vi "newSubject.vi"(8 "error in (no error)":errorcluster, 11 "reference in":refnum<class "Subject Controller.lvclass">) -> (0 "error out":errorcluster, 3 "reference out":refnum<class "Subject Controller.lvclass">)   [LabVIEW 2015, in "Subject Controller.lvclass"]
uses:
  Subject Controller.lvclass
  File Controller_llb/File Controller.lvclass
  APP/subject_class/subject.lvclass
  APP/subject_class/phase.ctl
  APP/subject_class/resultsType.ctl
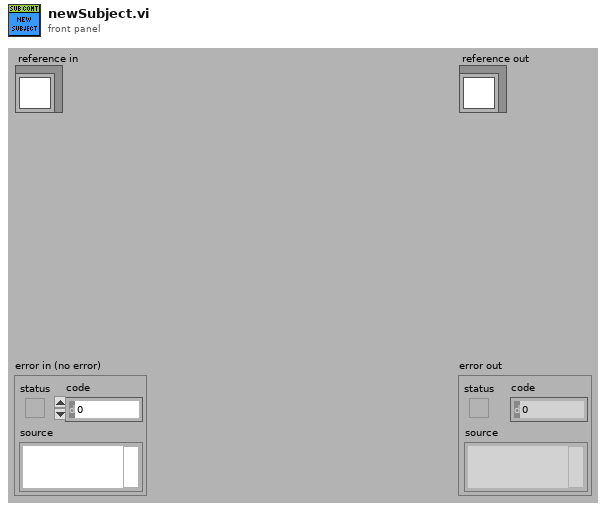
[diagram p1: front panel]
types:
  T1 = cluster{"Ve_warm":dbl[], "time_warm":dbl[], "name":string, "phase":dbl[], "VCO2":dbl[], "VO2":dbl[], "PetCO2":dbl[], "RQ":dbl[], "HR":dbl[], "Ve_warm_inter":dbl[], "time_warm_inter":dbl[], "Ve_exer":dbl[], "time_exer":dbl[], "Ve_exer_inter":dbl[], "time_exer_inter":dbl[], "Ve":dbl[], "time":dbl[], "Ve_exer_inter_filtered":dbl[], "Ve_warm_inter_filtered":dbl[]}
  T2 = typedef "Subject Controller.lvclass/ObjectAttributesRef.ctl" = refnum<data-value>
  T3 = typedef "Subject Controller.lvclass/ObjectAttributes.ctl" = cluster{"MyAttribute":dbl, "subject_controller_ref":refnum<class "Subject Controller.lvclass">, "file_controller_ref":refnum<class "File Controller.lvclass">, "subject_refs":refnum<class "subject.lvclass">[], "subjectIndex":i32, "file_type":T4}
  T4 = typedef "excelFile.lvclass/fileType.ctl" = enum16{"database", "CosmedTest"}
  T5 = typedef "subject.lvclass/resultsType.ctl" = enum16{"5L", "15%", "User Selection"}
  T6 = typedef "subject.lvclass/phase.ctl" = enum16{"warmUp", "userSelection", "Exercise"}
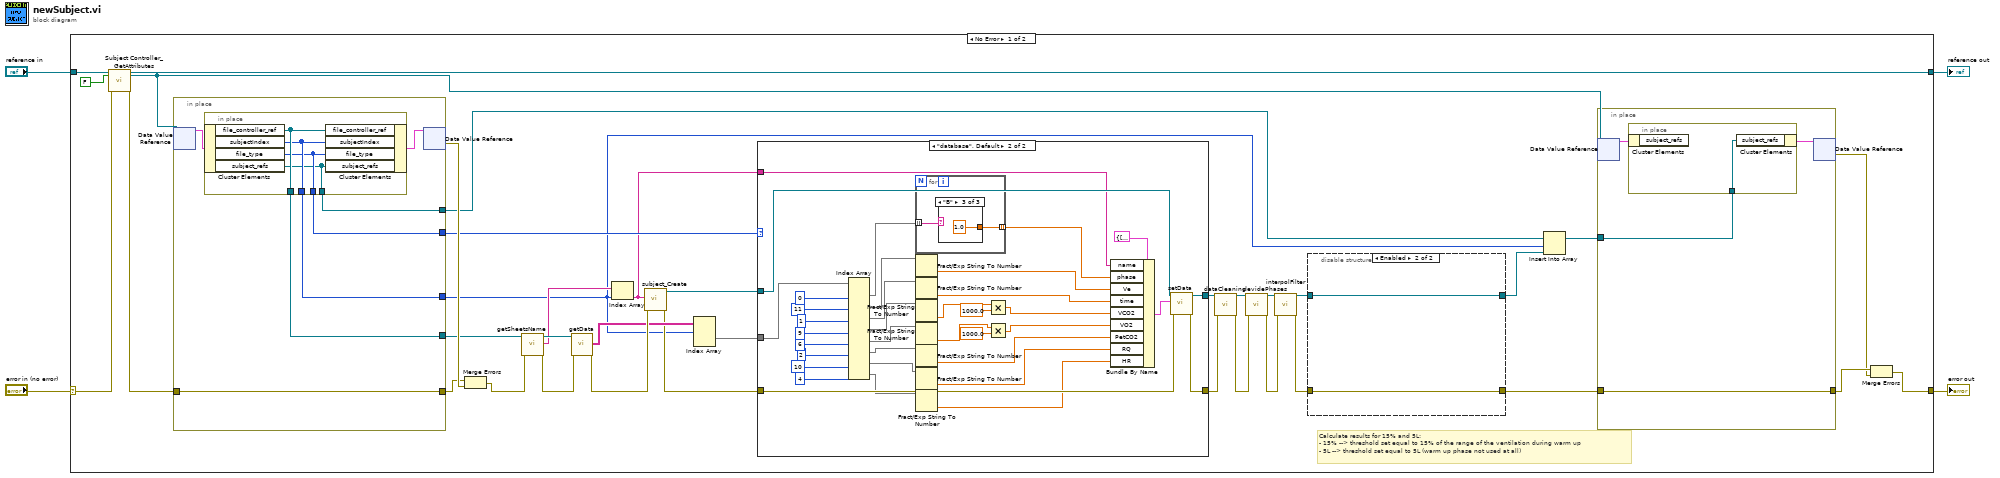
[diagram p0: block diagram]
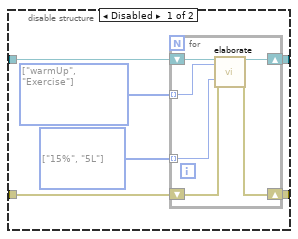
[diagram p2: hidden frame]
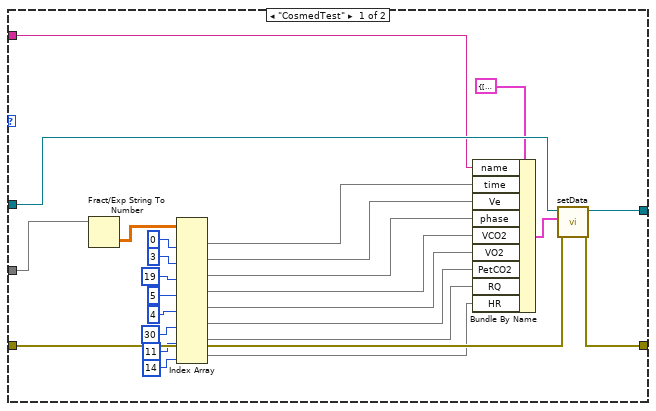
[diagram p3: hidden frame]
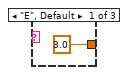
[diagram p4: hidden frame]
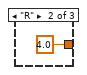
[diagram p5: hidden frame]
diagram:
  n1 = case shown="No Error" "error in (no error)" {
    selector: "error in (no error)" -> [w36 w138]
    tunnel: [w25 w138] -> w3
    tunnel: [w34 w137] -> w1
    tunnel: "reference in" -> [w38 w137]
    frame No Error {
      # "Calculate results for 15% and 5L:\n- 15% --> threshold set equal to 15% of the range of the ventilation during warm up\n- 5L --> threshold set equal to 5L (warm up phase not used at all)"
      n2 = call "Subject Controller_GetAttributes.vi"("reference in"=w38, "return data? (T)"=FALSE, "error in (no error)"=w36) -> ("reference out"=w34:refnum<class "Subject Controller.lvclass">, "attributes ref"=w17:T2, "error out"=w35:errorcluster)  [unwired: 13 in, 1 out]
      n3 = in-place {
        in-place-border: w35 -> [w130]
        in-place-border: [w130] -> w39
        in-place-border: [w129] -> w33
        in-place-border: [w128] -> w9
        in-place-border: [w127] -> w23
        in-place-border: [w126] -> w19
        n4 = in-place-dvr #1(w17) -> (w131:T3)  [unwired: 1 out]
        n5 = in-place {
          in-place-border: [w136] -> w129
          in-place-border: [w135] -> w128
          in-place-border: [w134] -> w127
          in-place-border: [w133] -> w126
          n6 = in-place-cluster #2(w131) -> ("file_controller_ref"=w136:refnum<class "File Controller.lvclass">, "subjectIndex"=w135:i32, "file_type"=w134:T4, "subject_refs"=w133:refnum<class "subject.lvclass">[])
          n7 = in-place-cluster #2("file_controller_ref"=w136, "subjectIndex"=w135, "file_type"=w134, "subject_refs"=w133) -> (w132:T3)
        }
        n8 = in-place-dvr #1(w132) -> (w40:errorcluster)  [unwired: 1 out]
      }
      n9 = Merge Errors(w39, w40) -> (w32:errorcluster)
      n10 = call "getSheetsName.vi"("reference in"=w33, "error in (no error)"=w32) -> ("reference out"=w31:refnum<class "File Controller.lvclass">, "sheetName"=w28:string[], "error out"=w30:errorcluster)  [unwired: 15 in]
      n11 = call "getData.vi"("reference in"=w31, "error in (no error)"=w30) -> ("data"=w24:string[][][], "error out"=w29:errorcluster)  [unwired: 15 in, 1 out]
      n12 = Index Array(array=w28, index=w9) -> (element=w16:string)
      n13 = call "subject_Create.vi"("error in (no error)"=w29, "name"=w16) -> ("error out"=w22:errorcluster, "reference out"=w20:refnum<class "subject.lvclass">)  [unwired: 8 in]
      n14 = Index Array(array=w24, index (dim 0)=w9) -> (element=w21:string[][])  [unwired: 2 in]
      n15 = case shown="\"database\", Default" w23 {
        tunnel: w22 -> [w79 w115]
        tunnel: [w78 w114] -> w14
        tunnel: w21 -> [w76 w111]
        tunnel: w20 -> [w74 w112]
        tunnel: [w77 w113] -> w15
        tunnel: w16 -> [w57 w82]
        frame "CosmedTest" {
          n16 = Fract/Exp String To Number(string=w76) -> (number=w75:dbl[][])  [unwired: 3 in, 1 out]
          n17 = Index Array(array=w75, index (col) #1=0 ("disabled index (col)"), index (col) #2=3 ("index (col)"), index (col) #3=19 ("index (col)"), index (col) #4=5 ("index (col)"), index (col) #5=4 ("index (col)"), index (col) #6=30 ("index (col)"), index (col) #7=11 ("index (col)"), index (col) #8=14 ("index (col)")) -> (element #1=w72:dbl[], element #2=w70:dbl[], element #3=w68:dbl[], element #4=w66:dbl[], element #5=w64:dbl[], element #6=w61:dbl[], element #7=w60:dbl[], element #8=w58:dbl[])  [unwired: 8 in]
          n18 = Bundle By Name(cluster=T1 {"Ve_warm"=[], "time_warm"=[], "name"="", "phase"=[], "VCO2"=[], "VO2"=[], "PetCO2"=[], "RQ"=[], "HR"=[], "Ve_warm_inter"=[], "time_warm_inter"=[], "Ve_exer"=[], "time_exer"=[], "Ve_exer_inter"=[], "time_exer_inter"=[], "Ve"=[], "time"=[], "Ve_exer_inter_filtered"=[], "Ve_warm_inter_filtered"=[]} ("data"), "name"=w57, "time"=w72, "Ve"=w70, "phase"=w68, "VCO2"=w66, "VO2"=w64, "PetCO2"=w61, "RQ"=w60, "HR"=w58) -> (w55:T1)
          n19 = call "setData.vi"("error in (no error)"=w79, "data"=w55, "reference in"=w74) -> ("error out"=w78:errorcluster, "reference out"=w77:refnum<class "subject.lvclass">)  [unwired: 7 in]
        }
        frame "database", Default {
          n20 = Index Array(array=w111, index (col) #1=0 ("disabled index (col)"), index (col) #2=11 ("index (col)"), index (col) #3=1 ("index (col)"), index (col) #4=9 ("index (col)"), index (col) #5=6 ("index (col)"), index (col) #6=2 ("index (col)"), index (col) #7=10 ("index (col)"), index (col) #8=4 ("index (col)")) -> (element #1=w109:string[], element #2=w107:string[], element #3=w105:string[], element #4=w101:string[], element #5=w95:string[], element #6=w91:string[], element #7=w87:string[], element #8=w85:string[])  [unwired: 8 in]
          n21 = for {
            tunnel: w109 -> [w117] mode=indexing
            tunnel: [w116] -> w108 mode=indexing
            n22 = case shown="\"B\"" w117 {
              tunnel: [3.0 4.0 1.0] -> w116
              frame "E", Default {
              }
              frame "R" {
              }
              frame "B" {
              }
            }
          }
          n23 = Fract/Exp String To Number(string=w107) -> (number=w106:dbl[])  [unwired: 3 in, 1 out]
          n24 = Fract/Exp String To Number(string=w105) -> (number=w104:dbl[])  [unwired: 3 in, 1 out]
          n25 = Fract/Exp String To Number(string=w101) -> (number=w100:dbl[])  [unwired: 3 in, 1 out]
          n26 = Fract/Exp String To Number(string=w95) -> (number=w94:dbl[])  [unwired: 3 in, 1 out]
          n27 = Fract/Exp String To Number(string=w91) -> (number=w90:dbl[])  [unwired: 3 in, 1 out]
          n28 = Fract/Exp String To Number(string=w87) -> (number=w86:dbl[])  [unwired: 3 in, 1 out]
          n29 = Fract/Exp String To Number(string=w85) -> (number=w84:dbl[])  [unwired: 3 in, 1 out]
          n30 = Multiply(x=w100, y=1000.0) -> (x*y=w98:dbl[])
          n31 = Multiply(x=w94, y=1000.0) -> (x*y=w93:dbl[])
          n32 = Bundle By Name(cluster=T1 {"Ve_warm"=[], "time_warm"=[], "name"="", "phase"=[], "VCO2"=[], "VO2"=[], "PetCO2"=[], "RQ"=[], "HR"=[], "Ve_warm_inter"=[], "time_warm_inter"=[], "Ve_exer"=[], "time_exer"=[], "Ve_exer_inter"=[], "time_exer_inter"=[], "Ve"=[], "time"=[], "Ve_exer_inter_filtered"=[], "Ve_warm_inter_filtered"=[]} ("data"), "name"=w82, "phase"=w108, "Ve"=w106, "time"=w104, "VCO2"=w98, "VO2"=w93, "PetCO2"=w90, "RQ"=w86, "HR"=w84) -> (w80:T1)
          n33 = call "setData.vi"("error in (no error)"=w115, "data"=w80, "reference in"=w112) -> ("error out"=w114:errorcluster, "reference out"=w113:refnum<class "subject.lvclass">)  [unwired: 7 in]
        }
      }
      n34 = call "dataCleaning.vi"("reference in"=w15, "error in (no error)"=w14) -> ("reference out"=w13:refnum<class "subject.lvclass">, "error out"=w11:errorcluster)  [unwired: 16 in]
      n35 = call "devidePhases.vi"("reference in"=w13, "error in (no error)"=w11) -> ("reference out"=w12:refnum<class "subject.lvclass">, "error out"=w10:errorcluster)  [unwired: 16 in]
      n36 = call "interpolFilter.vi"("reference in"=w12, "error in (no error)"=w10) -> ("reference out"=w8:refnum<class "subject.lvclass">, "error out"=w6:errorcluster)  [unwired: 16 in]
      n37 = disable-structure shown="Enabled" {
        disable-tunnel: w8 -> [w46 w54]
        disable-tunnel: [w45 w54] -> w7
        disable-tunnel: w6 -> [w44 w53]
        disable-tunnel: [w43 w53] -> w5
        frame Disabled {
          w41 = T5[] [enum."15%", enum."5L"] items=["5L", "15%", "User Selection"]
          w42 = T6[] [enum."warmUp", enum."Exercise"] items=["warmUp", "userSelection", "Exercise"]
          n38 = for {
            shift-right: [w51] -> w45
            shift-left: w46 -> [w52]
            shift-right: [w49] -> w43
            shift-left: w44 -> [w50]
            tunnel: w42 -> [w48] mode=indexing
            tunnel: w41 -> [w47] mode=indexing
            n39 = call "elaborate.vi"("reference in"=w52, "phase"=w48, "resultsType"=w47, "error in (no error)"=w50) -> ("reference out"=w51:refnum<class "subject.lvclass">, "error out"=w49:errorcluster)  [unwired: 14 in]
          }
        }
        frame Enabled {
        }
      }
      n40 = Insert Into Array(array=w19, index=w9, new element=w7) -> (w18:refnum<class "subject.lvclass">[])
      n41 = in-place {
        in-place-border: w5 -> [w122]
        in-place-border: [w122] -> w27
        in-place-border: w18 -> [w121]
        n42 = in-place-dvr #3(w17) -> (w123:T3)  [unwired: 1 out]
        n43 = in-place {
          in-place-border: w121 -> [w125]
          n44 = in-place-cluster #4(w123) -> ()  [unwired: 1 out]
          n45 = in-place-cluster #4("subject_refs"=w125) -> (w124:T3)
        }
        n46 = in-place-dvr #3(w124) -> (w26:errorcluster)  [unwired: 1 out]
      }
      n47 = Merge Errors(w27, w26) -> (w25:errorcluster)
    }
    frame Error {
    }
  }
  "error out" <- w3
  "reference out" <- w1
